vi "Configure Edge Trigger Source.vi"(6 "Trigger Slope (Positive)":string(combo)="POS", 8 "error in (no error)":errorcluster {"code" format="%.0x"}, 9 "Trigger Level (0.0 V)":dbl format="%^.2e", 10 "Trigger Source (Channel 1)":string(combo)="CHAN1", 11 "VISA Resource Name":refnum<visa-resource-name>) -> (0 "error out":errorcluster {"code" format="%.0x"}, 3 "VISA Resource Name Out":refnum<visa-resource-name>)   [LabVIEW 2011, in "Agilent 546XX Series.lvlib"]
doc: "This VI configures the edge trigger. An edge trigger occurs when the trigger signal passes through the voltage threshold that you specify with the Trigger Level control and has the slope that you specify with the Trigger Slope control. \n\nNotes:\n\n(1) This VI affects instrument behavior only if the Trigger Type is Edge Trigger. Call the ag546xx Configure Trigger VI to set the Trigger Type before you call this VI."
uses:
  Agilent 546XX Series.lvlib
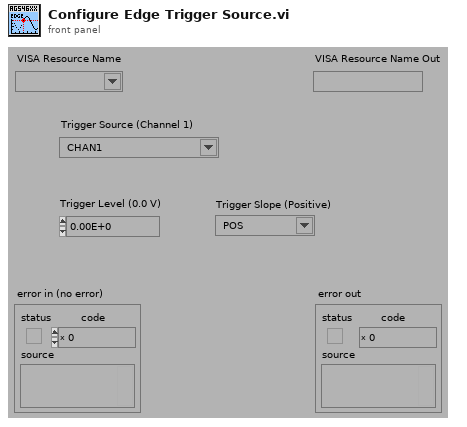
[diagram p1: front panel]
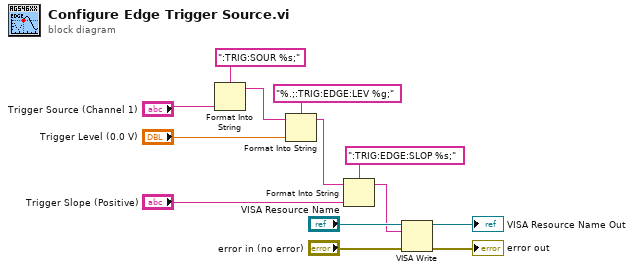
[diagram p0: block diagram]
diagram:
  n1 = Format Into String(format string=":TRIG:SOUR %s;", "Trigger Source (Channel 1)") -> (resulting string=w3:string)  [unwired: 2 in, 1 out]
  n2 = Format Into String(format string="%.;:TRIG:EDGE:LEV %g;", initial string=w3, "Trigger Level (0.0 V)") -> (resulting string=w4:string)  [unwired: 1 in, 1 out]
  n3 = Format Into String(format string=":TRIG:EDGE:SLOP %s;", initial string=w4, "Trigger Slope (Positive)") -> (resulting string=w2:string)  [unwired: 1 in, 1 out]
  n4 = VISA Write(VISA resource name="VISA Resource Name", write buffer=w2, error in (no error)="error in (no error)") -> (VISA resource name out=→"VISA Resource Name Out":refnum<visa-resource-name>, error out=→"error out":errorcluster)  [unwired: 1 out]
